vi "Database Testing.vi"() -> ()   [LabVIEW 2018]
doc: "The T1 Parametric testing application performs parametric testing of T1 signals. The T1 signal is a 1.544 Mb/s pulsed digital signal formed by multiplexing 24 voice channels. Each channel is sampled at 8000 samples/sec. Each sample is then converted to 8 bits using Pulse Coded Multiplexing. The 24 channels are then time-division multiplexed. Each frame, which corresponds to one sampling period, contains 192 bits ( 8 times 24) plus one bit for frame synchronization. Since frames occur at 8000 times per second, the bit rate is 1.544 Mb/s\n\nThis application performs the following parametric tests on T1 signals:\n\n1. Mask Test: Compares T1 signals with standard masks. The type of masks that are supported are ITU G.703 mask, EIA/TIA 547 and ANSI T1.102. The graph shows the mask in grey, the actual signal in green and failures as red squares. A boolean indicates whether the signal passed or failed the mask test and the indicator Number of Hits shows the number of times the signal did not pass the mask test.\n\n2. Measure T1 signal amplitude : Measures the amplitude of the T1 signal. The peak amplitude is displayed in the indicator Measured Amplitude.\n\n3. Measure T1 signal frequency : Measures the frequency of the T1 signal. The signal frequency in MHz is displayed in the indicator Measured Frequency."
uses:
  <vilib>/addons/database/Connection.llb/DB Tools Open Connec (Path).vi
  <vilib>/addons/database/NI_Database_API.lvlib
panel:
  in  "Stop":bool
  in  "Launch Retrieval VI":bool
  in  "Launch Logging VI":bool
  # "Overview: Demonstrates a sample application that logs data to a database and retrieves data from the database.\nRequirements: Database Connectivity Toolkit\nInstructions:\n1. Run the VI.\n2. Click Launch Logging VI to launch a VI that logs data to a database.\n3. Click Launch Retrieval VI to launch a VI that retrieves data from the database.\n4. Click Stop to stop the VI."
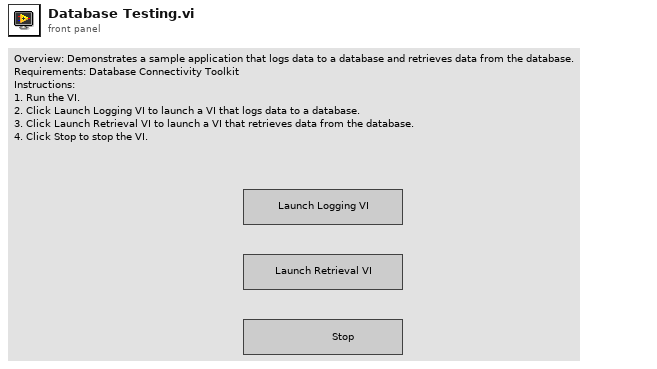
[diagram p1: front panel]
types:
  T1 = typedef "NI_Database_API.lvlib/Conn ObjectReference.ctl" = refnum<k1>
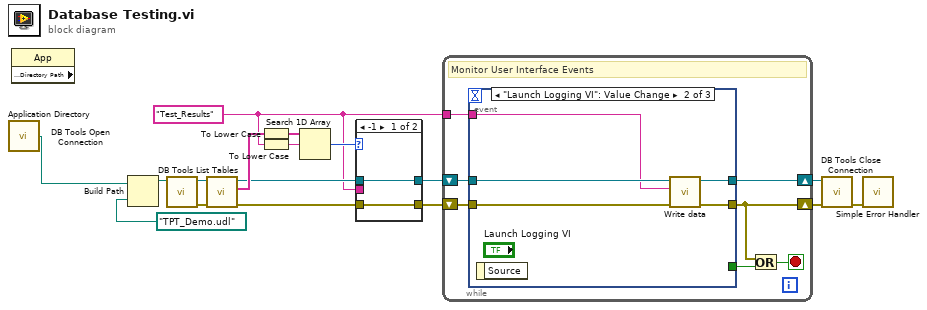
[diagram p0: block diagram]
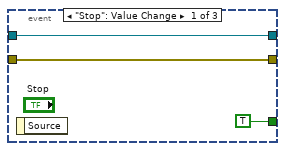
[diagram p2: hidden frame]
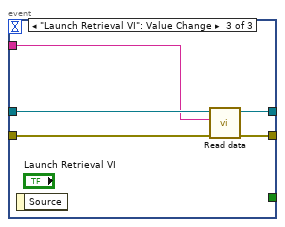
[diagram p3: hidden frame]
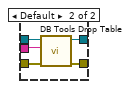
[diagram p4: hidden frame]
diagram:
  w2 = "Test_Results" ("element")
  n1 = call <vilib>:"Application Directory.vi"() -> ("Application Directory"=w1:path)
  n2 = property class="App" props=["Application:Directory Path"]() -> ()  [unwired: 2 in, 3 out]
  n3 = Build Path(base path=w1, name or relative path=path "TPT_Demo.udl" ("Application:Directory Path")) -> (appended path=w13:path)
  n4 = call-poly <vilib>:"DB Tools Open Connection.vi"("connection information"=w13) -> ("error out"=w16:errorcluster, "connection reference"=w15:T1)  [unwired: 7 in]
  n5 = call <vilib>:"DB Tools List Tables.vi"("error in (no error)"=w16, "connection reference"=w15) -> ("error out"=w12:errorcluster, "tables"=w17:string[], "connection reference out"=w11:T1)  [unwired: 3 in]
  n6 = To Lower Case(string=w17) -> (all lower case string=w4:string[])
  n7 = To Lower Case(string=w2) -> (all lower case string=w3:string)
  n8 = Search 1D Array(1D array=w4, element=w3) -> (index of element=w5:i32)  [unwired: 1 in]
  n9 = case shown="-1" w5 {
    tunnel: w11 -> [w19 w23]
    tunnel: w12 -> [w18 w24]
    tunnel: [w19 w22] -> w8
    tunnel: [w18 w21] -> w9
    tunnel: w2 -> [_ w20]
    frame -1 {
    }
    frame Default {
      n10 = call <vilib>:"DB Tools Drop Table.vi"("error in (no error)"=w24, "table"=w20, "connection reference"=w23) -> ("error out"=w21:errorcluster, "connection reference out"=w22:T1)  [unwired: 5 in]
    }
  }
  n11 = while {
    shift-left: w9 -> [w30]
    shift-right: [w27] -> w6
    shift-left: w8 -> [w29]
    shift-right: [w28] -> w7
    tunnel: w2 -> [w25]
    stop <- w31 stop-if-true
    # "Monitor User Interface Events"
    n12 = event shown="[1] \"Launch Logging VI\": Value Change" {
      selector: _ -> [_ _ _]
      dyn-events: _ -> [_ _ _]
      timeout: _ -> [_ _ _]
      tunnel: w30 -> [w34 w38 w43]
      tunnel: [w34 w35 w41] -> w27
      tunnel: w29 -> [w33 w37 w44]
      tunnel: [w33 w39 w42] -> w28
      tunnel: [TRUE _ _] -> w26
      tunnel: w25 -> [_ w36 w40]
      event "Stop": Value Change {
        n13 = event-data() -> ()  [unwired: 1 in, 1 out]
      }
      event "Launch Logging VI": Value Change {
        n14 = event-data() -> ()  [unwired: 1 in, 1 out]
        n15 = call "Write data.vi"("error in (no error)"=w38, "table name"=w36, "connection reference"=w37) -> ("error out"=w35:errorcluster, "connection reference out"=w39:T1)  [unwired: 7 in]
      }
      event "Launch Retrieval VI": Value Change {
        n16 = event-data() -> ()  [unwired: 1 in, 1 out]
        n17 = call "Read data.vi"("error in (no error)"=w43, "table name"=w40, "connection reference"=w44) -> ("error out"=w41:errorcluster, "connection reference out"=w42:T1)  [unwired: 7 in]
      }
    }
    n18 = Or(x=w27, y=w26) -> (x .or. y?=w31:bool)
  }
  n19 = call <vilib>:"DB Tools Close Connection.vi"("error in (no error)"=w6, "connection reference"=w7) -> ("error out"=w10:errorcluster)  [unwired: 5 in]
  n20 = call <vilib>:"Simple Error Handler.vi"("error in (no error)"=w10) -> ()  [unwired: 4 in, 5 out]
